vi "Clear Channel Mapping.vi"(11 "Destination":refnum<k24>) -> ()   [LabVIEW 2019, in "Software Multi-Plex System Explorer.lvlib"]
uses:
  Software Multi-Plex System Explorer.lvlib
  NationalInstruments.VeriStand.SystemStorage
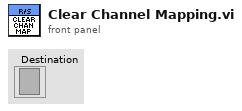
[diagram p1: front panel]
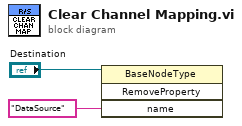
[diagram p0: block diagram]
diagram:
  n1 = invoke class="BaseNodeType" method="RemoveProperty"(reference="Destination", "name"="DataSource") -> ()  [unwired: 2 in, 4 out]
